vi "tls write.vi"(8 "error in":errorcluster, 10 "data":string, 11 "tls context":u64) -> (0 "error out":errorcluster, 3 "error response":i32)   [LabVIEW 2016, in "lv tls dll.lvlib"]
uses:
  lv tls dll.lvlib
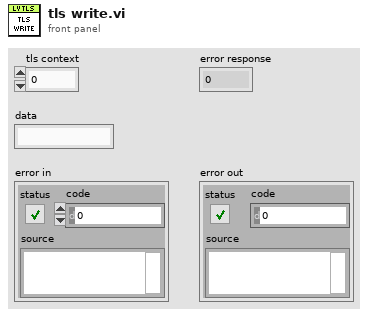
[diagram p1: front panel]
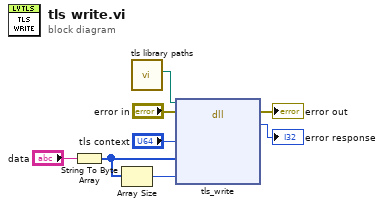
[diagram p0: block diagram]
diagram:
  n1 = String To Byte Array(string="data") -> (unsigned byte array=w3:u8[])
  n2 = Array Size(array=w3) -> (size(s)=w4:i32)
  n3 = call "tls library paths.vi"() -> ("libtls"=w8:path)  [unwired: 8 in, 3 out]
  n4 = dll-call lib="C:/Users/IEUser/Desktop/tlssimple/libtls-15.dll" fn="tls_write"(path in=w8, error in="error in", "context"="tls context", "buf"=w3, "buflen"=w4) -> (error out=→"error out":errorcluster, "err"=→"error response":i32)  [unwired: 4 in, 1 out]
